vi "Get Result as Timestamp from DateTime.vi"(8 "error in (no error)":errorcluster, 10 "Use Milliseconds":bool=TRUE, 11 "Parameter in":refnum<class "Parameter.lvclass">) -> (0 "error out":errorcluster, 2 "Result":timestamp, 3 "Parameter out":refnum<class "Parameter.lvclass">)   [LabVIEW 2023, in "HAF.lvlib" / "Parameter.lvclass"]
doc: "Returns the Raw Result converted to a Timestamp with date and time. Raw Result must be in Date Time order. If Raw Result is not compatible then an incorrect conversion may occur or an error raised."
uses:
  Parameter.lvclass
  HAF.lvlib
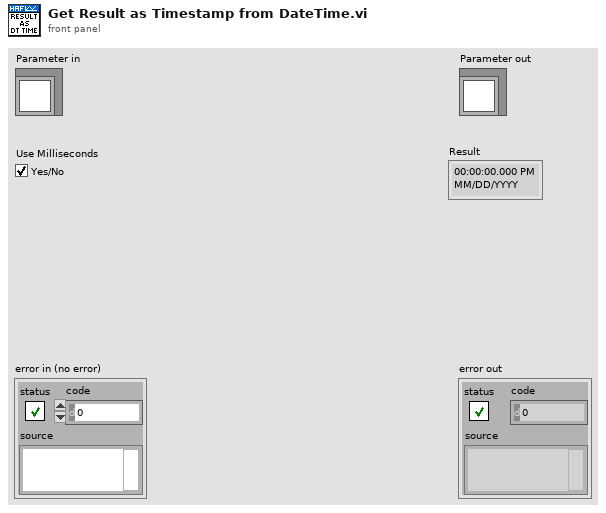
[diagram p1: front panel]
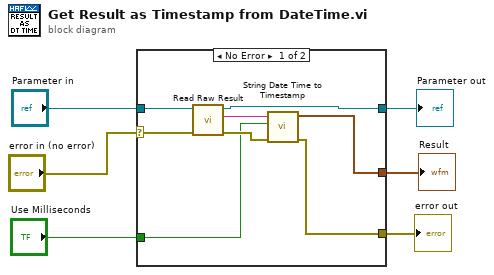
[diagram p0: block diagram]
diagram:
  n1 = case shown="No Error" "error in (no error)" {
    selector: "error in (no error)" -> [w13 w16]
    tunnel: [w7 w16] -> w5
    tunnel: [w9 w15] -> w3
    tunnel: "Parameter in" -> [w14 w15]
    tunnel: "Use Milliseconds" -> [w10 _]
    tunnel: [w8 _] -> w1
    frame No Error {
      n2 = call-dynamic "Read Raw Result.vi"("error in (no error)"=w13, "Parameter in"=w14) -> ("error out"=w11:errorcluster, "Raw Result"=w12:string, "Parameter out"=w9:refnum<class "Parameter.lvclass">)  [unwired: 7 in]
      n3 = call "String Date Time to Timestamp.vi"("error in (no error)"=w11, "Use milliseconds"=w10, "String to Convert"=w12) -> ("error out"=w7:errorcluster, "Timestamp Value"=w8:timestamp)  [unwired: 7 in]
    }
    frame Error {
    }
  }
  "error out" <- w5
  "Parameter out" <- w3
  "Result" <- w1
